vi "RMS_ACV_No_DC_filter.vi"(9 "# of samples":dbl, 11 "Data IN":dbl[](array[numeric])) -> (3 "VRMS":dbl)   [LabVIEW 2012]
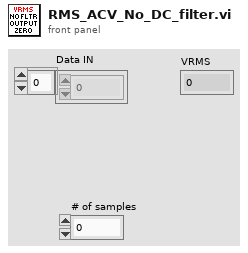
[diagram p1: front panel]
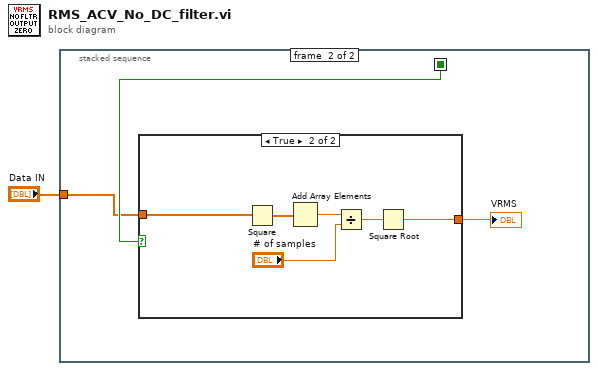
[diagram p0: block diagram]
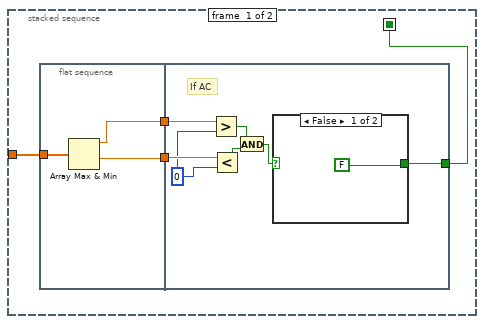
[diagram p2: hidden frame]
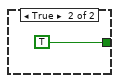
[diagram p3: hidden frame]
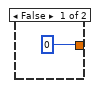
[diagram p4: hidden frame]
diagram:
  n1 = stacked-sequence {
    seq-local: [w5 _] -> [_ w20]
    tunnel: "Data IN" -> [w2 w18]
    frame #0 {
      n2 = flat-sequence {
        tunnel: [w8] -> w4
        tunnel: [w7] -> w3
        tunnel: w2 -> [w6]
        tunnel: [w15] -> w5
        tunnel: w4 -> [w14]
        tunnel: w3 -> [w12]
        frame #0 {
          n3 = Array Max & Min(array=w6) -> (max value=w7:dbl, min value=w8:dbl)  [unwired: 2 out]
        }
        frame #1 {
          w13 = 0
          # "If AC"
          n4 = Greater?(x=w12, y=w13) -> (0:w10:bool)
          n5 = Less?(x=w14, y=w13) -> (x < y?=w9:bool)
          n6 = And(x=w10, y=w9) -> (x .and. y?=w11:bool)
          n7 = case shown="False" w11 {
            tunnel: [FALSE TRUE] -> w15
            frame False {
            }
            frame True {
            }
          }
        }
      }
    }
    frame #1 {
      n8 = case shown="True" w20 {
        tunnel: [0 w23] -> w19
        tunnel: w18 -> [_ w22]
        frame False {
        }
        frame True {
          n9 = Square(x=w22) -> (x^2=w25:dbl[])
          n10 = Add Array Elements(numeric array=w25) -> (sum=w26:dbl)
          n11 = Divide(x=w26, y="# of samples") -> (x/y=w27:dbl)
          n12 = Square Root(x=w27) -> (sqrt(x)=w23:dbl)
        }
      }
      "VRMS" <- w19
    }
  }
